vi "Set Digital Filter [FRD].vi"(7 "Micropulse # In":i32, 8 "error in (no error)":errorcluster, 9 "Low Pass Filter":T1 caption="LPF", 10 "High Pass Filter":T2 caption="HPF", 11 "Test Number":u32) -> (0 "error out":errorcluster, 5 "Micropulse # Out":i32)   [LabVIEW 2026, in "MicroPulse_Driver.lvlib"]
doc: "One of six high pass and six low pass digital filters can be selected. By default the digital filters are disabled. To enable the use, an FRD -1 1 1 command must be sent. This then enables an internal gate extension to ensure the correct operation of the filters for the entire user inspection gate.\nTo disable the gate extension FRD -1 0 0 should be sent.\n\nParameters:\n<Tn> : Test number. An integer value from 0 to the maximum number of tests (default maximum is 1279 tests).\nTn = 0 for all conventional tests. If the S extension is used it applies to all tests in the sweep number specified: 1-32, 0 = all sweeps.\n\n<High pass filter > :\n0 = none\n1 = 0.7MHz High-pass\n2 = 1.5MHz High-pass\n3 = 4.0MHz High-pass\n4 = 7.5MHz High-pass\n5 = 10.0MHz High-pass\n6 = Use defined\n\n<Low pass filter > :\n0 = none\n1 = 1.8MHz Low-pass\n2 = 3.0MHz Low-pass\n3 = 6.0MHz Low-pass\n4 = 8.0MHz Low-pass\n5 = 12MHz Low-pass\n6 = Use defined\n\nExample:\nFRD 1 3 4 : Sets test 1 to a 4 – 8 MHz bandpass filter\n\nSystem Compatibility:\nIncompatible for FMC tests (AMP 13 mode)"
uses:
  MicroPulse_Driver.lvlib
  <instrlib>/MicroPulse/Public/Data/Datatypes/MP - high pass filter.ctl
  <instrlib>/MicroPulse/Public/Data/Datatypes/MP - low pass filter.ctl
  <instrlib>/MicroPulse/Public/Data/Datatypes/MP - instrument type.ctl
  Private/MP-Registry Action-Enum.ctl
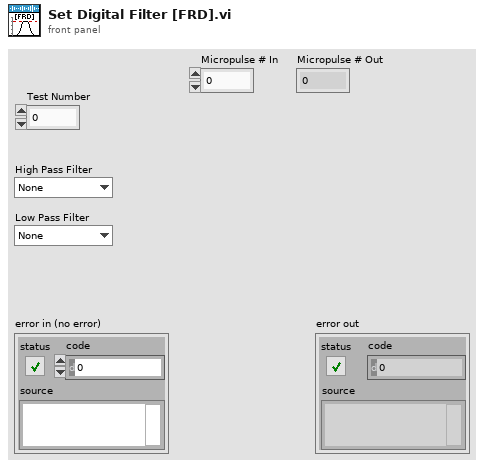
[diagram p1: front panel]
types:
  T1 = typedef "MicroPulse_Driver.lvlib/MP - low pass filter.ctl" = enum16{"None", "1.8MHz", "3.0MHz", "6.0MHz", "8.0MHz", "12.0MHz", "User Defined"}
  T2 = typedef "MicroPulse_Driver.lvlib/MP - high pass filter.ctl" = enum16{"None", "0.7MHz", "1.5MHz", "4.0MHz", "7.5MHz", "10.0MHz", "User Defined"}
  T3 = typedef "MicroPulse_Driver.lvlib/MP - instrument type.ctl" = enum16{"MicroPulse 5", "LT1", "LT2", "LTPA", "MPLT", "MicroPulse 6", "PipeScanner", "<MicroPulse>", "Micropulse 4", "Simulated Data"}
  T4 = typedef "MicroPulse_Driver.lvlib/MP-Registry Data-Cluster.ctl" = cluster{"Instrument Type":T3, "Serial #":u64, "Sample Frequency":T5, "dt (us)":dbl, "DOF":T6, "Material Velocity":dbl, "Asynch Reads":T7, "NUM of Tests":u32, "System Details":T8, "Gates":T10[], "Encoders":T17[], "CMD LUT":variant, "Command List":string}
  T5 = typedef "MicroPulse_Driver.lvlib/MP - sample frequency.ctl" = enum16{"Use Default", "200MHz (LT2 only)", "100MHz", "50MHz", "25MHz", "10MHz"}
  T6 = typedef "MicroPulse_Driver.lvlib/MP - data output format.ctl" = enum16{"", "8-bit Mode", "10-bit Mode", "12-bit Mode", "16-bit Mode", "8-bit Log Mode", "12-bit Packed Mode"}
  T7 = typedef "MicroPulse_Driver.lvlib/MP - asynch read mode.ctl" = enum16{"Disabled", "Enabled"}
  T8 = typedef "MicroPulse_Driver.lvlib/MP - general system status.ctl" = cluster{"System Type":T3, "Serial No.":u64, "Channels":cluster{"Conv":u8, "PA":u16, "Extra":u32}, "Sample Frequency":cluster{"Default":u8, "Actual":u8}, "Software Versions":string, "Data Output Format":cluster{"Default":T6, "Actual":T6}, "Temperatures":cluster{"System":u8, "Processor":u8, "Slave Sys":u8, "Slave Proc":u8}, "Tx Buffer Size":u32, "System Error":string, "No. of Cards":u8, "DAC Gain":i16, "Uptimes":cluster{"since Power":u32, "since RSTS":u32, "since SRST":u32}, "Voltages":cluster{"Nominal":dbl, "Measured":dbl, "Difference":dbl}[], "Interface Cards":T9[]}
  T9 = typedef "MicroPulse_Driver.lvlib/MP - interface card status.ctl" = cluster{"Status":u8, "Map":u8, "Board - T":u8, "FPGA - T":u8, "PAIF Status":string, "Version":string}
  T10 = typedef "MicroPulse_Driver.lvlib/MP - Registry Gates.ctl" = cluster{"Display Gate":T11, "ETM Mode":T12, "Echo Gate":T13, "Insp Gates":T14[]}
  T11 = typedef "MicroPulse_Driver.lvlib/MP - display gate.ctl" = cluster{"Start":dbl, "Length":dbl}
  T12 = typedef "MicroPulse_Driver.lvlib/MP - echo gate mode.ctl" = enum16{"Echo Trigger OFF", "Echo Gate Display Mode", "Echo Trigger ON", "Multi Gate or FMC Mode", "Reserved", "PA - Echo Trigger ON"}
  T13 = typedef "MicroPulse_Driver.lvlib/MP - echo gate parameters.ctl" = cluster{"Start (us)":dbl, "Length (us)":dbl, "Threshold":u16, "Colour":u32}
  T14 = typedef "MicroPulse_Driver.lvlib/MP - multigate inspection gate parameters.ctl" = cluster{"Start (us)":dbl, "Length (us)":dbl, "Threshold":u16, "Enabled?":bool, "Max # Peaks":u16, "Hysteresis":T15, "Mode":T16, "Inverted?":bool, "Colour ":u32}
  T15 = typedef "MicroPulse_Driver.lvlib/MP - hysteresis level.ctl" = enum16{"None", "3dB", "6dB", "9dB", "12dB"}
  T16 = typedef "MicroPulse_Driver.lvlib/MP - multigate mode.ctl" = enum16{"1st Peak in Gate", "Largest Peak In Gate", "All Peaks In Gate", "1st Threshold Crossing"}
  T17 = typedef "MicroPulse_Driver.lvlib/MP - encoder settings.ctl" = cluster{"Encoder Type":T18, "Counts/mm":u32, "Enable Termination?":bool, "Multiplier":u32, "Backlash Period (s)":dbl, "Encoder Filter":u32}
  T18 = typedef "MicroPulse_Driver.lvlib/MP - encoder type.ctl" = enum16{"Quadrature", "Step/Direction"}
  T19 = typedef "MicroPulse_Driver.lvlib/TCP config.ctl" = cluster{"Connection ID":refnum<k5>, "IP address":string, "host port":u16, "OC timeout":i32, "Read timeout":i32, "Write timeout":i32}
  T20 = typedef "MicroPulse_Driver.lvlib/MP-Registry Action-Enum.ctl" = enum16{"Read", "Add Test", "Add Command", "Add Gate Command", "Add Encoder Command", "Clear Command  List", "Set Registry", "Set System Details", "Set DOF", "Set Velocity", "Disable Asynch Reads", "Enable Asynch Reads", "Add Connection", "Disconnect", "Shutdown"}
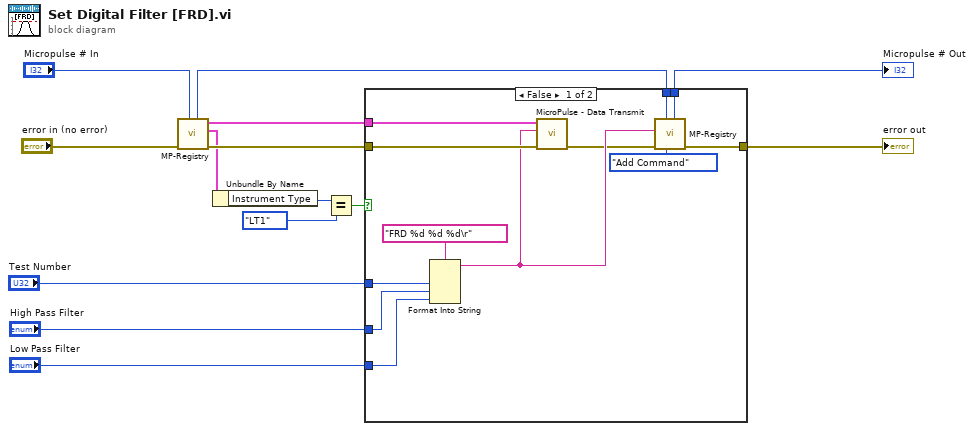
[diagram p0: block diagram]
diagram:
  n1 = call "MP-Registry.vi"("Micropulse # In"="Micropulse # In", "error in (no error)"="error in (no error)") -> ("error out"=w9:errorcluster, "Micropulse Data"=w4:T4, "TCP config"=w8:T19, "Micropulse # Out"=w7:i32)  [unwired: 6 in]
  n2 = Unbundle By Name(w4) -> ("Instrument Type"=w3:T3)
  n3 = Equal?(x=w3, y=MP_-_instrument_type."LT1") -> (x = y?=w1:bool)
  n4 = case shown="False" w1 {
    tunnel: "Test Number" -> [w26 _]
    tunnel: [w25 w28] -> w11
    tunnel: [w24 w27] -> w10
    tunnel: w9 -> [w23 w28]
    tunnel: w8 -> [w22 _]
    tunnel: w7 -> [w18 w27]
    tunnel: "High Pass Filter" -> [w16 _]
    tunnel: "Low Pass Filter" -> [w15 _]
    frame False {
      n5 = Format Into String(format string="FRD %d %d %d\r", w26, w16, w15) -> (resulting string=w21:string)  [unwired: 2 in, 1 out]
      n6 = call "MicroPulse - Data Transmit.vi"("error in (no error)"=w23, "data"=w21, "TCP config"=w22) -> ("error out"=w19:errorcluster)  [unwired: 6 in, 2 out]
      n7 = call "MP-Registry.vi"("Action"=MP-Registry_Action-Enum."Add Command", "Micropulse # In"=w18, "error in (no error)"=w19, "Data in"=w21) -> ("error out"=w25:errorcluster, "Micropulse # Out"=w24:i32)  [unwired: 4 in, 2 out]
    }
    frame True {
      # "LT1 does not have digital filters"
    }
  }
  "error out" <- w11
  "Micropulse # Out" <- w10
